vi "5224A.vi"(8 "error in (no error)":errorcluster caption="错误输入（无错误）", 10 "vnaPortName":refnum<visa-resource-name>, 11 "5224A输入":refnum<class "5224A.lvclass">) -> (0 "error out":errorcluster caption="错误输出", 3 "5224A输出":refnum<class "5224A.lvclass">)   [LabVIEW 2011, in "5224A.lvclass"]
uses:
  5224A.lvclass
  5224A.lvclass/5224A.ctl
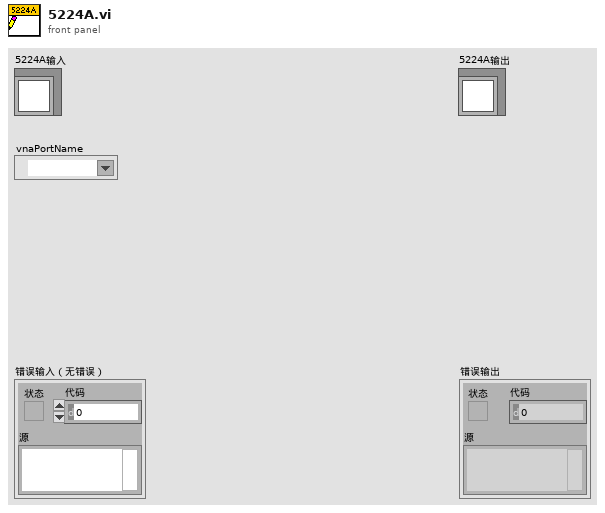
[diagram p1: front panel]
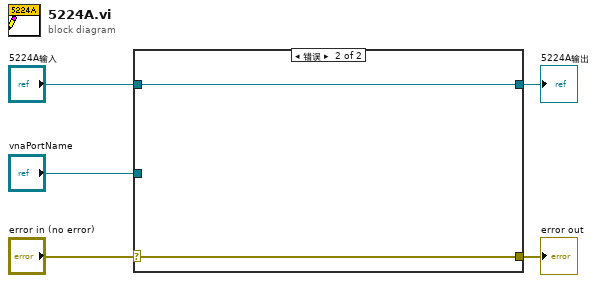
[diagram p0: block diagram]
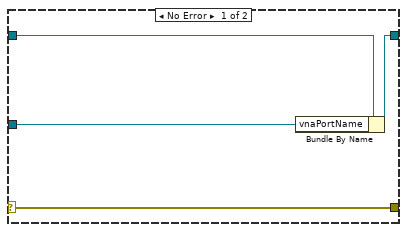
[diagram p2: hidden frame]
diagram:
  n1 = case shown="错误" "error in (no error)" {
    selector: "error in (no error)" -> [w9 w10]
    tunnel: [w9 w10] -> w4
    tunnel: [w7 w11] -> w2
    tunnel: "5224A输入" -> [w8 w11]
    tunnel: "vnaPortName" -> [w6 _]
    frame No Error {
      n2 = Bundle By Name(cluster=w8, "vnaPortName"=w6) -> (w7:refnum<class "5224A.lvclass">)
    }
    frame Error {
    }
  }
  "error out" <- w4
  "5224A输出" <- w2
